vi "Read Trim Settings Configuration File.vi"(11 "FIle_Name":string="Trim Limits_KGD") -> (3 "Trim_Settings_Array 2":T1=[{"Test_Name"="ODFT_Trim", "Target"=1.9, "Reg_Add_0X00"=81, "Data_LSB"=4, "Data_Length"=4, "Settings"=[8, 9, 10, 11, 12, 13, 14, 15, 0, 1, 2, 3, 4, 5, 6, 7], "MSB_Reg_Add_0X00"=0, "Data_MSB"=0}, {"Test_Name"="HV_Trim", "Target"=39.0, "Reg_Add_0X00"=81, "Data_LSB"=0, "Data_Length"=4, "Settings"=[7, 6, 5, 4, 3, 2, 1, 0, 15, 14, 13, 12, 11, 10, 9, 8], "MSB_Reg_Add_0X00"=0, "Data_MSB"=0}, {"Test_Name"="Freq_Trim", "Target"=20.0, "Reg_Add_0X00"=80, "Data_LSB"=0, "Data_Length"=4, "Settings"=[0, 1, 2, 3, 4, 5, 6, 7, 8, 9, 10, 11, 12, 13, 14, 15], "MSB_Reg_Add_0X00"=0, "Data_MSB"=0}] {"MSB_Reg_Add_0X00" format="%.0x"; "Reg_Add_0X00" format="%.0x"})   [LabVIEW 2013]
uses:
  Controls/Trim_Config_Settings_Array.ctl
  Controls/Trim_Config_Settings.ctl
  <vilib>/Utility/file.llb/Read From Spreadsheet File (string).vi
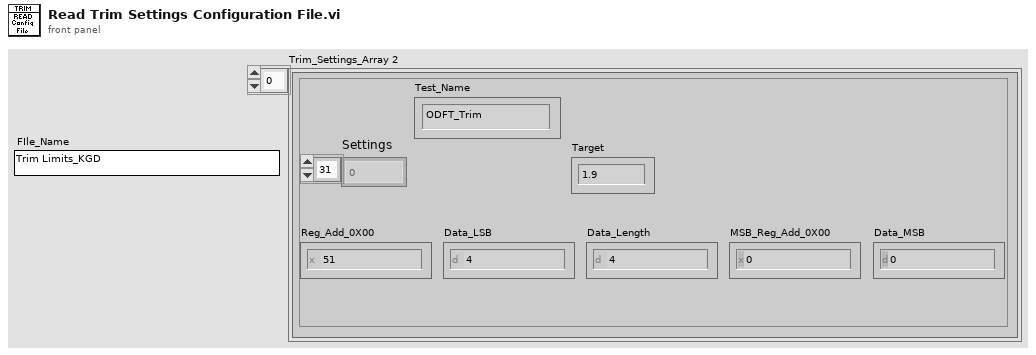
[diagram p1: front panel]
types:
  T1 = typedef "Trim_Config_Settings_Array.ctl" = T2[]
  T2 = typedef "Trim_Config_Settings.ctl" = cluster{"Test_Name":string, "Target":dbl, "Reg_Add_0X00":u8, "Data_LSB":u8, "Data_Length":u8, "Settings":u8[], "MSB_Reg_Add_0X00":u8, "Data_MSB":u8}
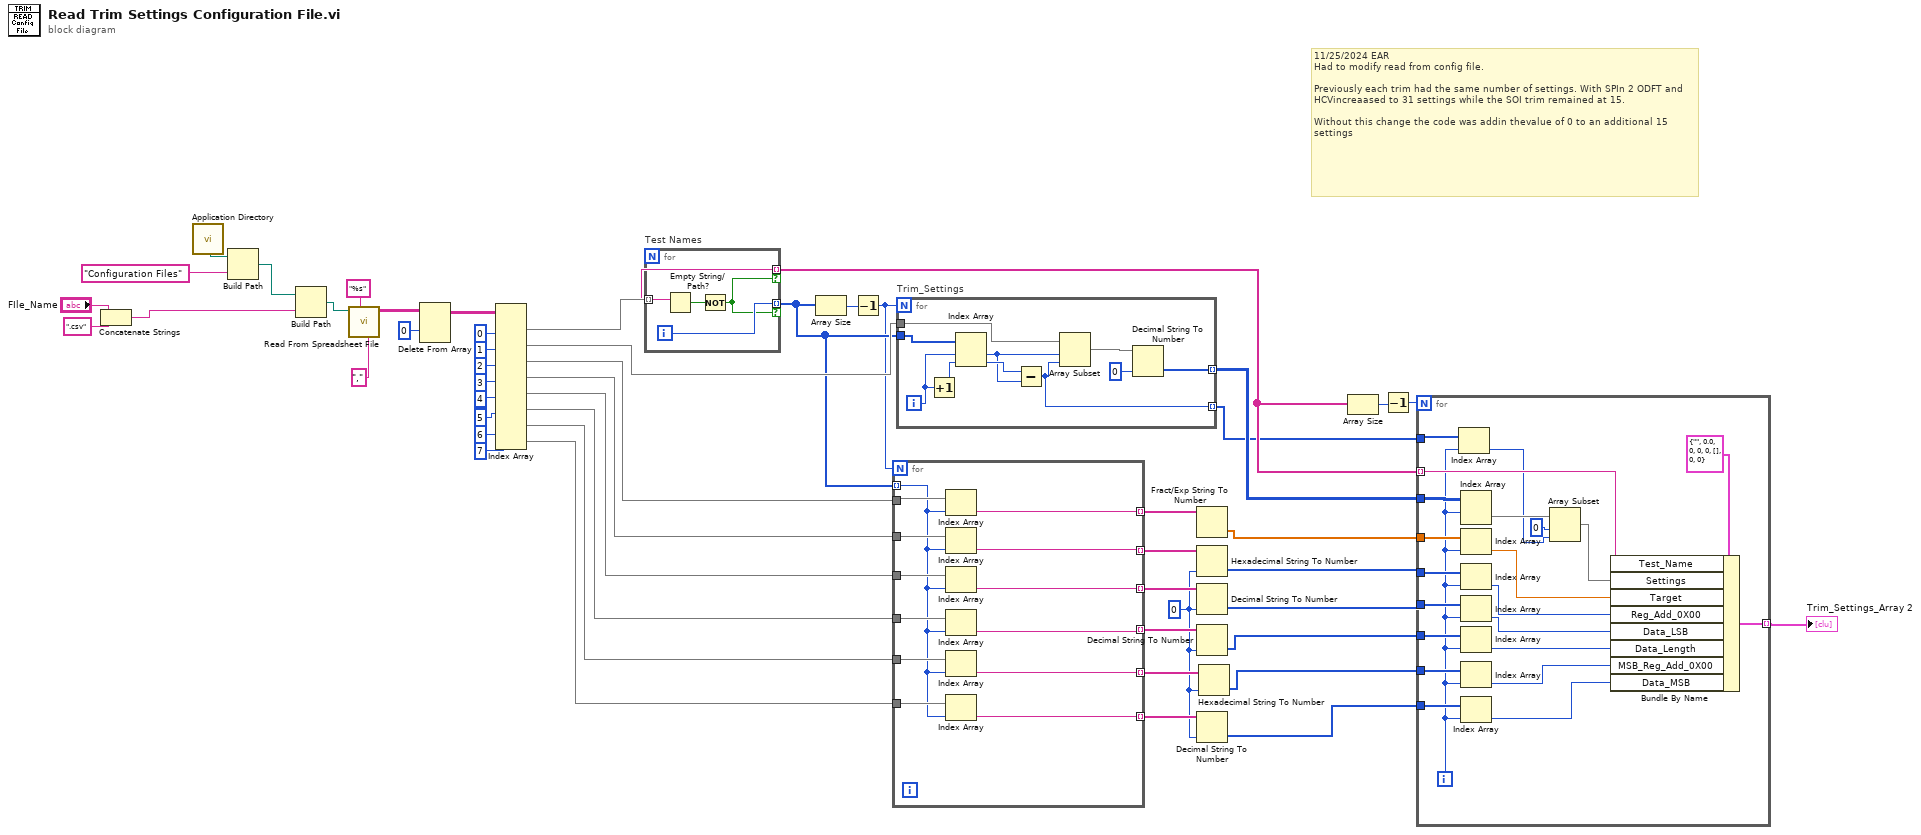
[diagram p0: block diagram]
diagram:
  w5 = u8 0 ("default (0 U32)")
  # "11/25/2024 EAR\nHad to modify read from config file.\n\nPreviously each trim had the same number of settings. With SPIn 2 ODFT and HCVincreaased to 31 settings while the SOI trim remained at 15. \n\nWithout this change the code was addin thevalue of 0 to an additional 15 settings"
  n1 = Concatenate Strings("FIle_Name", ".csv" ("string")) -> (w16:string)
  n2 = call <vilib>:"Application Directory.vi"() -> ("Application Directory"=w3:path)
  n3 = Build Path(base path=w3, name or relative path="Configuration Files") -> (appended path=w1:path)
  n4 = Build Path(base path=w1, name or relative path=w16) -> (appended path=w15:path)
  n5 = call-poly <vilib>:"Read From Spreadsheet File.vi"("delimiter (\\t)"="," ("delimiter (\\t)"), "format (%s)"="%s", "file path (dialog if empty)"=w15) -> ("all rows"=w48:string[][])  [unwired: 4 in, 4 out]
  n6 = Delete From Array(array=w48, index (row)=0) -> (array with subset deleted=w46:string[][])  [unwired: 2 in, 1 out]
  n7 = Index Array(array=w46, index (col) #1=0 ("disabled index (col)"), index (col) #2=1 ("index (col)"), index (col) #3=2 ("index (col)"), index (col) #4=3 ("disabled index (col)"), index (col) #5=4 ("index (col)"), index (col) #6=5 ("index (col)"), index (col) #7=6 ("index (col)"), index (col) #8=7 ("index (col)")) -> (element #1=w40:string[], element #2=w39:string[], element #3=w34:string[], element #4=w31:string[], element #5=w30:string[], element #6=w29:string[], element #7=w11:string[], element #8=w10:string[])  [unwired: 8 in]
  n8 = for "Test Names" {
    tunnel: w40 -> [w52] mode=indexing
    tunnel: [w54] -> w33 mode=indexing if=w51
    tunnel: [w52] -> w35 mode=indexing if=w51
    i -> [w54]
    n9 = Empty String/Path?(string/path=w52) -> (empty?=w53:bool)
    n10 = Not(x=w53) -> (.not. x?=w51:bool)
  }
  n11 = Array Size(array=w33) -> (size(s)=w38:i32)
  n12 = Decrement(x=w38) -> (x-1=w32:i32)
  n13 = for {
    N: w32 -> [_]
    tunnel: w34 -> [w67]
    tunnel: w33 -> [w55] mode=indexing
    tunnel: [w66] -> w22 mode=indexing
    tunnel: w31 -> [w65]
    tunnel: [w64] -> w21 mode=indexing
    tunnel: w30 -> [w63]
    tunnel: [w62] -> w26 mode=indexing
    tunnel: [w61] -> w25 mode=indexing
    tunnel: w29 -> [w60]
    tunnel: w11 -> [w59]
    tunnel: w10 -> [w58]
    tunnel: [w57] -> w7 mode=indexing
    tunnel: [w56] -> w9 mode=indexing
    n14 = Index Array(array=w67, index=w55) -> (element=w66:string)
    n15 = Index Array(array=w65, index=w55) -> (element=w64:string)
    n16 = Index Array(array=w63, index=w55) -> (element=w62:string)
    n17 = Index Array(array=w60, index=w55) -> (element=w61:string)
    n18 = Index Array(array=w59, index=w55) -> (element=w57:string)
    n19 = Index Array(array=w58, index=w55) -> (element=w56:string)
  }
  n20 = for "Trim_Settings" {
    N: w32 -> [_]
    tunnel: w33 -> [w77]
    tunnel: w39 -> [w74]
    tunnel: [w69] -> w27 mode=indexing
    tunnel: [w68] -> w14 mode=indexing
    i -> [w76]
    n21 = Increment(x=w76) -> (x+1=w75:i32)
    n22 = Index Array(array=w77, index #1=w76, index #2=w75) -> (element #1=w72:i32, element #2=w73:i32)
    n23 = Subtract(x=w73, y=w72) -> (x-y=w68:i32)
    n24 = Array Subset(array=w74, index=w72, length=w68) -> (w70:string[])
    n25 = Decimal String To Number(string=w70, default (0L)=i8 0 ("default (0 I32)")) -> (number=w69:i8[])  [unwired: 1 in, 1 out]
  }
  n26 = Fract/Exp String To Number(string=w22) -> (number=w19:dbl[])  [unwired: 3 in, 1 out]
  n27 = Hexadecimal String To Number(string=w21, default (0uL)=w5) -> (number=w20:u8[])  [unwired: 1 in, 1 out]
  n28 = Decimal String To Number(string=w26, default (0L)=w5) -> (number=w24:u8[])  [unwired: 1 in, 1 out]
  n29 = Decimal String To Number(string=w25, default (0L)=w5) -> (number=w23:u8[])  [unwired: 1 in, 1 out]
  n30 = Decimal String To Number(string=w9, default (0L)=w5) -> (number=w8:u8[])  [unwired: 1 in, 1 out]
  n31 = Hexadecimal String To Number(string=w7, default (0uL)=w5) -> (number=w6:u8[])  [unwired: 1 in, 1 out]
  n32 = Array Size(array=w35) -> (size(s)=w37:i32)
  n33 = Decrement(x=w37) -> (x-1=w36:i32)
  n34 = for {
    N: w36 -> [_]
    tunnel: w35 -> [w99] mode=indexing
    tunnel: w27 -> [w98]
    tunnel: w20 -> [w97]
    tunnel: w24 -> [w95]
    tunnel: w23 -> [w96]
    tunnel: [w91] -> w4 mode=indexing
    tunnel: w19 -> [w90]
    tunnel: w14 -> [w86]
    tunnel: w6 -> [w83]
    tunnel: w8 -> [w82]
    i -> [w79]
    n35 = Index Array(array=w86, index=w79) -> (element=w85:i32)
    n36 = Index Array(array=w98, index (row)=w79) -> (element=w88:i8[])  [unwired: 1 in]
    n37 = Index Array(array=w90, index=w79) -> (element=w89:dbl)
    n38 = Index Array(array=w97, index=w79) -> (element=w94:u8)
    n39 = Index Array(array=w95, index=w79) -> (element=w93:u8)
    n40 = Index Array(array=w96, index=w79) -> (element=w92:u8)
    n41 = Index Array(array=w83, index=w79) -> (element=w81:u8)
    n42 = Index Array(array=w82, index=w79) -> (element=w80:u8)
    n43 = Array Subset(array=w88, index=0, length=w85) -> (w87:i8[])
    n44 = Bundle By Name(cluster=T2 {"Test_Name"="", "Target"=0.0, "Reg_Add_0X00"=0, "Data_LSB"=0, "Data_Length"=0, "Settings"=[], "MSB_Reg_Add_0X00"=0, "Data_MSB"=0} ("Trim_Settings"), "Test_Name"=w99, "Settings"=w87, "Target"=w89, "Reg_Add_0X00"=w94, "Data_LSB"=w93, "Data_Length"=w92, "MSB_Reg_Add_0X00"=w81, "Data_MSB"=w80) -> (w91:T2)
  }
  "Trim_Settings_Array 2" <- w4
